vi "Jiaxin_Goto.vi"(8 "error in (no error)":errorcluster, 9 "Abs Position Registers":u16[](array[numeric]), 10 "Channel":i32, 11 "MB Serial Master:MB_Master":refnum<class "MB_Master.lvclass">) -> (0 "error out":errorcluster, 3 "MB Serial Master:MB_Master":refnum<class "MB_Master.lvclass">)   [LabVIEW 2023, in "Jiaxin_Stepper_Controller.lvlib" / "Jiaxin_Stepper.lvclass"]
uses:
  Jiaxin_Stepper/Jiaxin_Stepper.lvclass
  <vilib>/Plasmionique/MB Master/MB_Master/MB_Master.lvclass
  Jiaxin_Stepper/Jiaxin_Stepper.lvclass/Jiaxin_Stepper.ctl
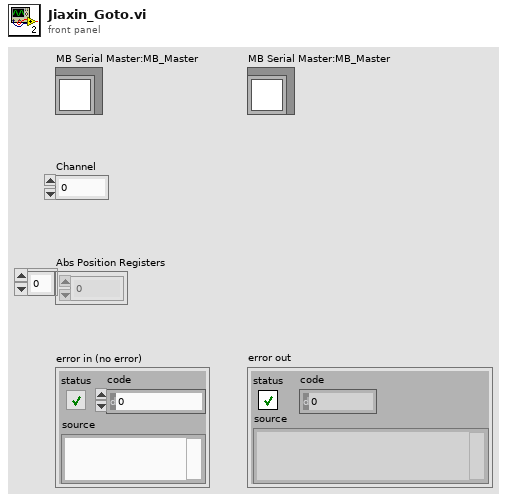
[diagram p1: front panel]
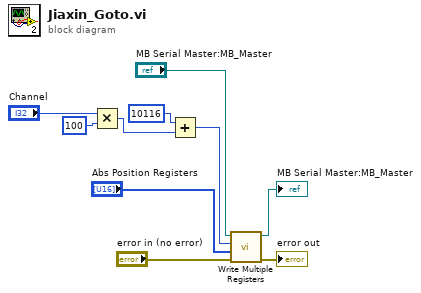
[diagram p0: block diagram]
diagram:
  n1 = Multiply(x="Channel", y=100) -> (x*y=w3:i32)
  n2 = Add(x=10116, y=w3) -> (x+y=w5:i32)
  n3 = call <vilib>:"Write Multiple Registers.vi"("error in (no error)"="error in (no error)", "values"="Abs Position Registers", "starting address"=w5, "MB session in"="MB Serial Master:MB_Master") -> ("error out"=→"error out":errorcluster, "MB session out"=→"MB Serial Master:MB_Master":refnum<class "MB_Master.lvclass">)  [unwired: 6 in]
